vi "Kinect MVMT.vi"() -> ()   [LabVIEW 2011]
panel:
  out "Timestamp":i32
  out "Diff Image":T1(plugin-control)
  out "x-y":u32
  out "Image":T1(plugin-control)
  in  "stop":bool
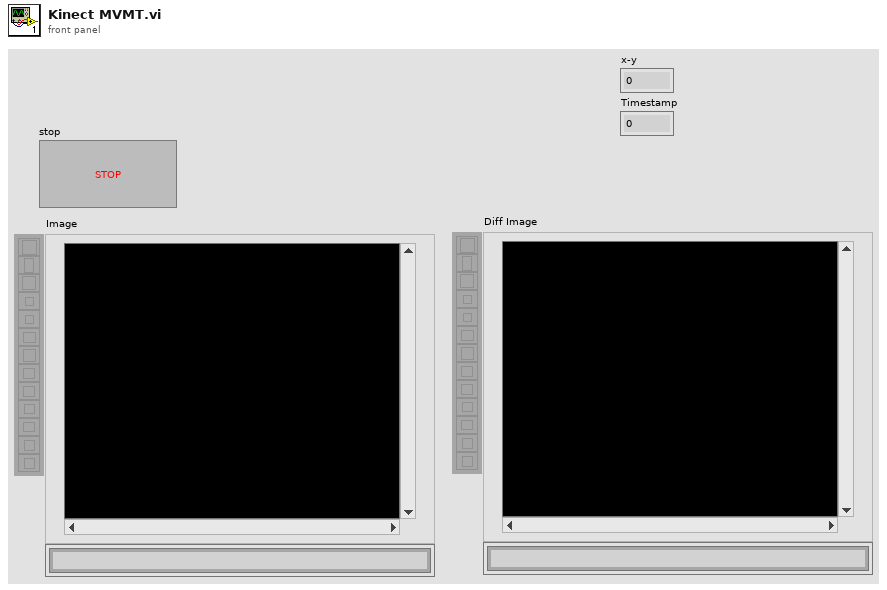
[diagram p1: front panel]
types:
  T1 = typedef "IMAQ Image.ctl" = refnum<image>
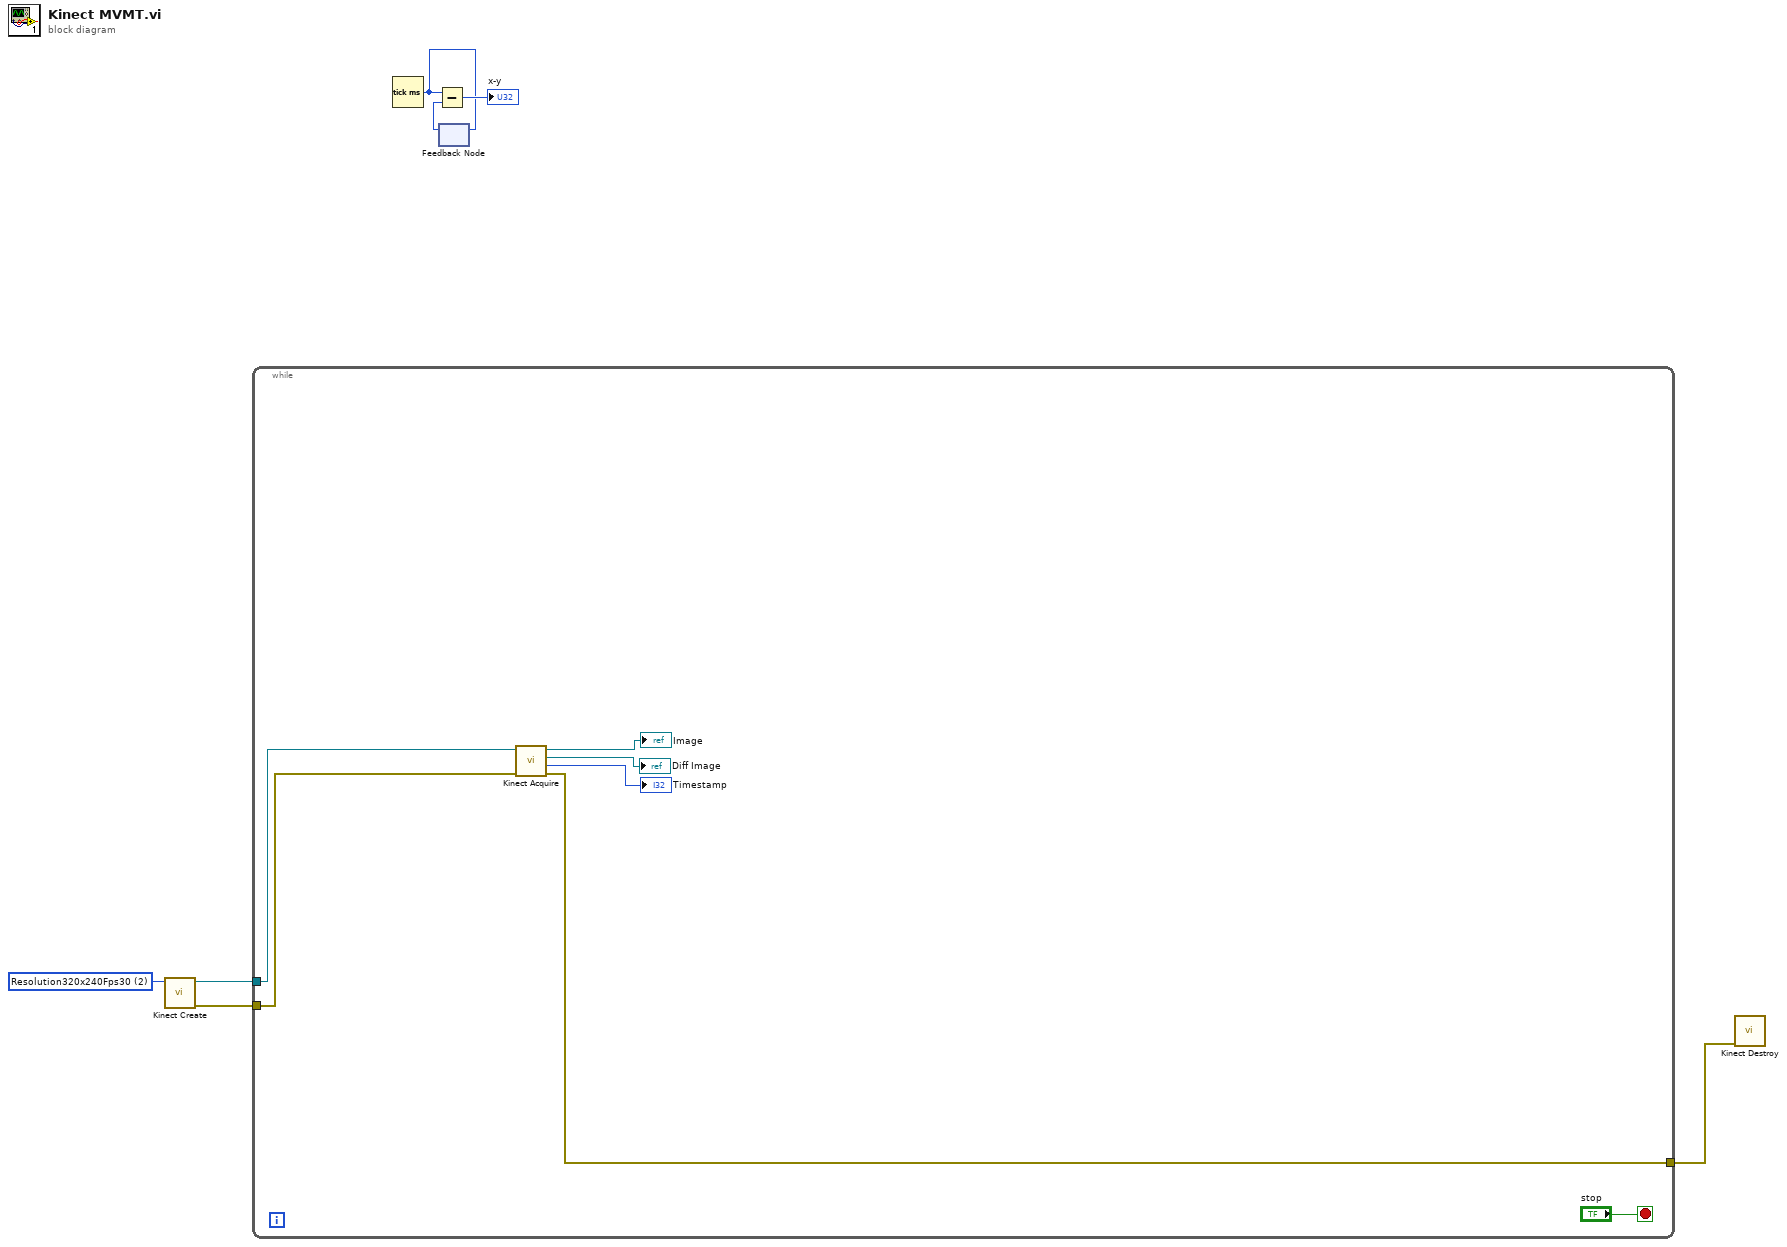
[diagram p0: block diagram]
diagram:
  w7 = 2 items=["Undefined", "Resolution640x480Fps30", "Resolution320x240Fps30", "Resolution80x60Fps30"] ("Depth Format")
  n1 = call "Kinect Create.vi"("Depth Format"=w7) -> ("error out"=w1:errorcluster, "queue out"=w5:refnum<queue>)  [unwired: 9 in]
  n2 = while {
    tunnel: w5 -> [w8]
    tunnel: [w10] -> w6
    tunnel: w1 -> [w11]
    stop <- "stop" stop-if-true
    n3 = call "Kinect Acquire.vi"("error in"=w11, "Queue in"=w8) -> ("error out"=w10:errorcluster, "Timestamp"=→"Timestamp":i32, "Difference\nImage"=→"Diff Image":T1, "Image Out"=→"Image":T1)  [unwired: 6 in]
  }
  n4 = Tick Count (ms)() -> (millisecond timer value=w2:u32)
  n5 = feedback #1() -> (w3:u32)  [unwired: 1 in]
  n6 = Subtract(x=w2, y=w3) -> (x-y=→"x-y":u32)
  n7 = feedback-in #1(w2) -> ()
  n8 = call "Kinect Destroy.vi"("error in"=w6) -> ()  [unwired: 10 in, 1 out]
